vi "DT_With_Multiplexer.vi"() -> ()   [LabVIEW 2012]
doc: "This vi will take data with multiple DT boxes for an arbitrary number of channels either differentially or single ended, depending upon how you have wired the boxes up."
uses:
  Globals/Meas_global.vi
panel:
  out "Waveform Graph":dbl[][](graph)
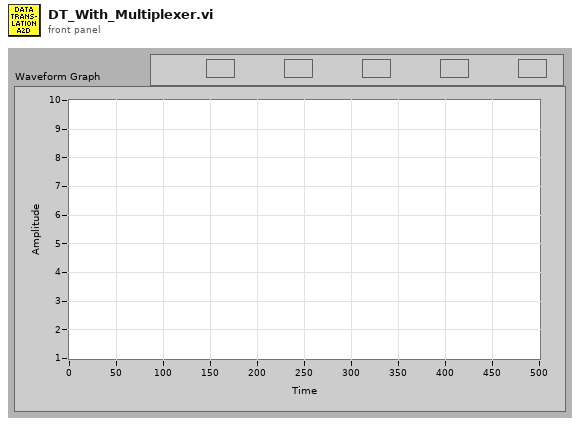
[diagram p1: front panel]
types:
  T1 = typedef "Trigger_Mode.ctl" = enum16{"Free Running", "Start on Trigger", "Trigger Every Block", "Trigger Every Sample"}
  T2 = typedef "LDA_Setup.ctl" = cluster{"dimensions":enum16{"1D", "2D"}, "Analogue Freq Multiplier":dbl}
  T3 = typedef "Ch_and_Spans.ctl" = cluster{"high limit (10V)":sgl, "low limit (-10V)":sgl, "Ch No":i16, "Var name":string, "Use Latest Calib":bool}
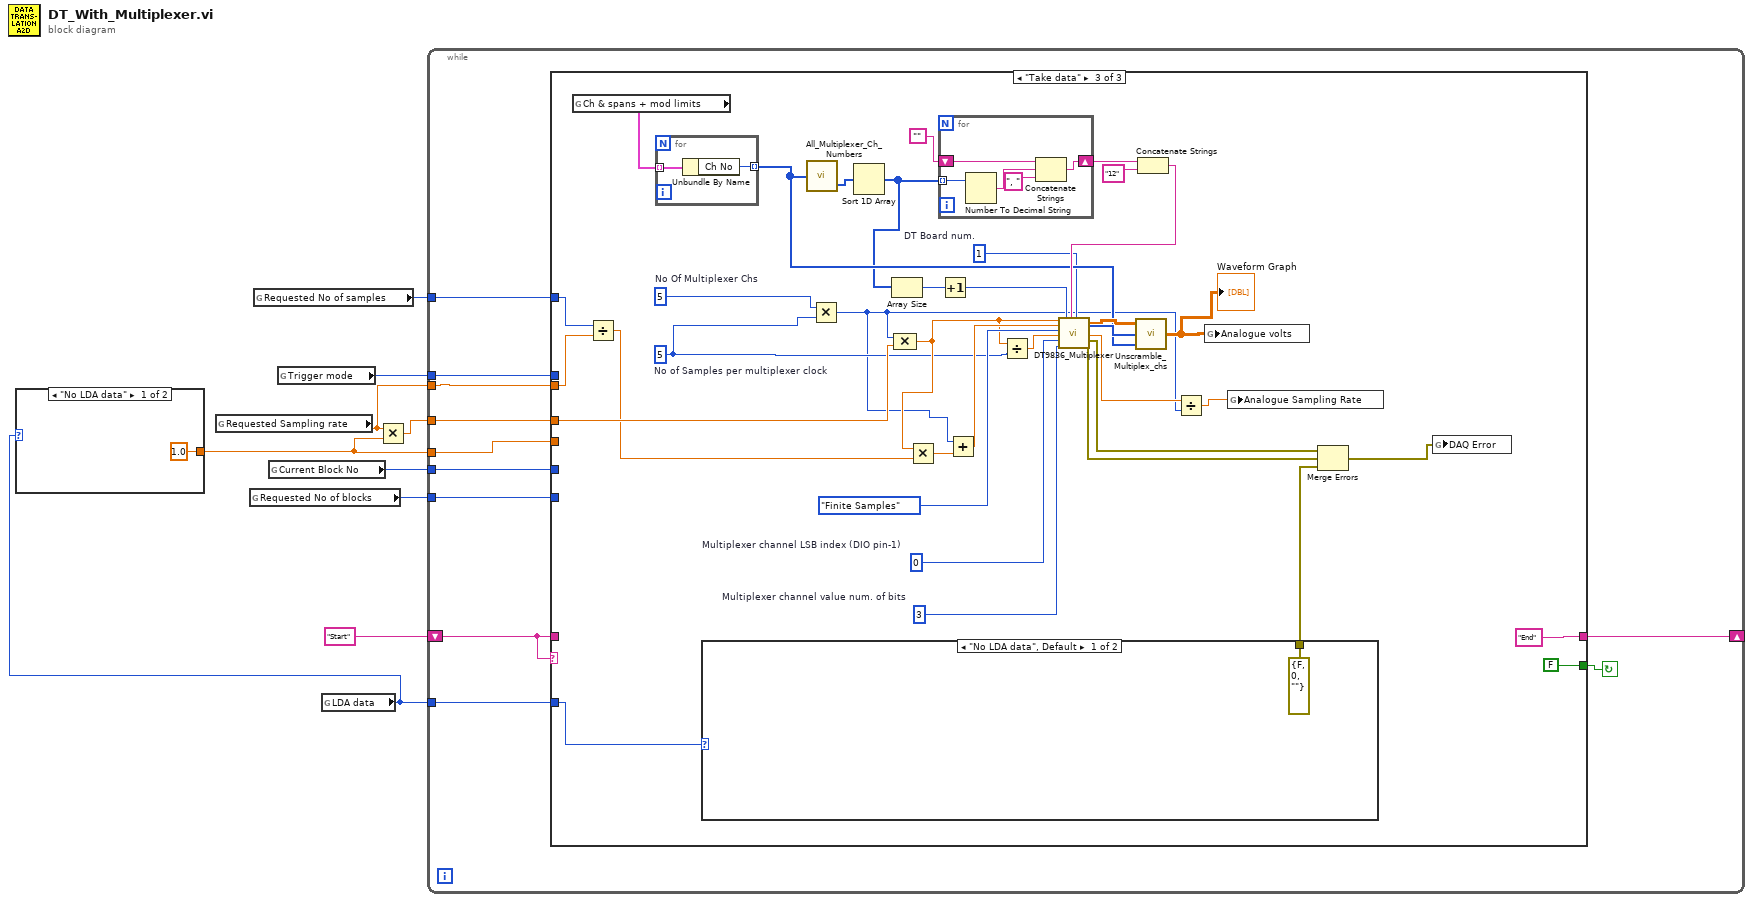
[diagram p0: block diagram]
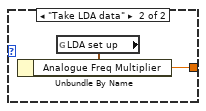
[diagram p2: hidden frame]
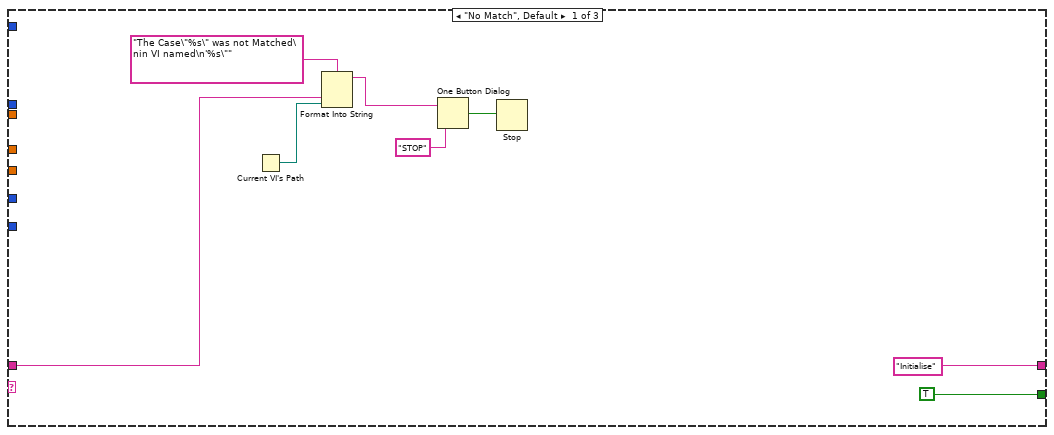
[diagram p3: hidden frame]
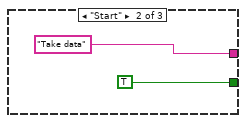
[diagram p4: hidden frame]
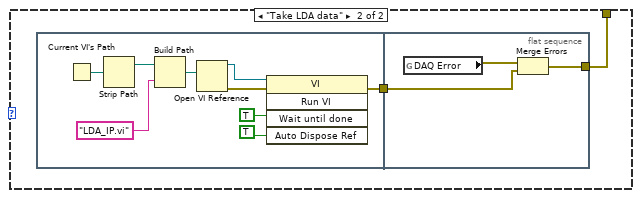
[diagram p5: hidden frame]
diagram:
  n1 = global read "Meas_global.vi" "Requested Sampling rate"() -> (w4:dbl)
  n2 = global read "Meas_global.vi" "Requested No of blocks"() -> (w3:i32)
  n3 = global read "Meas_global.vi" "Requested No of samples"() -> (w8:i32)
  n4 = global read "Meas_global.vi" "Current Block No"() -> (w6:i32)
  n5 = global read "Meas_global.vi" "Trigger mode"() -> (w7:T1)
  n6 = global read "Meas_global.vi" "LDA data"() -> (w1:enum16{"No LDA data", "Take LDA data"})
  n7 = case shown="\"No LDA data\"" w1 {
    tunnel: [1.0 ("Analogue Freq Multiplier") w11] -> w2
    frame "No LDA data" {
    }
    frame "Take LDA data" {
      n8 = global read "Meas_global.vi" "LDA set up"() -> (w12:T2)
      n9 = Unbundle By Name(w12) -> ("Analogue Freq Multiplier"=w11:dbl)
    }
  }
  n10 = Multiply(x=w4, y=w2) -> (x*y=w5:dbl)
  n11 = while {
    shift-left: "Start" -> [w22]
    shift-right: [w23] -> _
    tunnel: w5 -> [w21]
    tunnel: w8 -> [w20]
    tunnel: w6 -> [w19]
    tunnel: w7 -> [w17]
    tunnel: w1 -> [w16]
    tunnel: w2 -> [w15]
    tunnel: w4 -> [w14]
    tunnel: w3 -> [w13]
    stop <- w18 continue-if-true
    n12 = case shown="\"Take data\"" w22 {
      tunnel: ["Initialise" "Take data" "End"] -> w23
      tunnel: w22 -> [w27 _ _]
      tunnel: w21 -> [_ _ w62]
      tunnel: w20 -> [_ _ w61]
      tunnel: w19 -> [_ _ _]
      tunnel: [TRUE TRUE FALSE] -> w18
      tunnel: w17 -> [_ _ _]
      tunnel: w16 -> [_ _ w68]
      tunnel: w15 -> [_ _ _]
      tunnel: w14 -> [_ _ w39]
      tunnel: w13 -> [_ _ _]
      frame "No Match", Default {
        n13 = Current VI's Path() -> (path=w26:path)
        n14 = Format Into String(format string="The Case\"%s\" was not Matched\nin VI named\n'%s\"" ("Format String"), w27, w26) -> (resulting string=w30:string)  [unwired: 2 in, 1 out]
        n15 = One Button Dialog(message=w30, button name ("OK")="STOP") -> (true=w28:bool)
        n16 = Stop(stop? (T)=w28) -> ()
      }
      frame "Start" {
      }
      frame "Take data" {
        w44 = 3  # Multiplexer channel value num. of bits
        w45 = 0  # Multiplexer channel LSB index (DIO pin-1)
        w46 = u32 1  # DT Board num.
        w54 = 5  # No of Samples per multiplexer clock
        w58 = 5  # No Of Multiplexer Chs
        n17 = global read "Meas_global.vi" "Ch & spans + mod limits"() -> (w67:T3[])
        n18 = Divide(x=w61, y=w39) -> (x/y=w60:dbl)
        n19 = for {
          tunnel: w67 -> [w77] mode=indexing
          tunnel: [w76] -> w49 mode=indexing
          n20 = Unbundle By Name(w77) -> ("Ch No"=w76:i16)
        }
        n21 = case shown="\"No LDA data\", Default" w68 {
          tunnel: [errorcluster {"status"=FALSE, "code"=0, "source"=""} ("error IO") w79] -> w41
          frame "No LDA data", Default {
          }
          frame "Take LDA data" {
            n22 = flat-sequence {
              tunnel: [w81] -> w80
              tunnel: w80 -> [w91]
              tunnel: [w90] -> w79
              frame #0 {
                n23 = Current VI's Path() -> (path=w83:path)
                n24 = Strip Path(path=w83) -> (stripped path=w82:path)  [unwired: 1 out]
                n25 = Build Path(base path=w82, name or relative path="LDA_IP.vi") -> (appended path=w84:path)
                n26 = Open VI Reference(vi path=w84) -> (vi reference=w87:refnum<vi>, error out=w88:errorcluster)  [unwired: 5 in]
                n27 = invoke class="VI" method="Run VI"(reference=w87, error in=w88, "Wait until done"=TRUE ("Wait Until Done"), "Auto Dispose Ref"=TRUE ("Wait until done")) -> (error out=w81:errorcluster)  [unwired: 1 in, 4 out]
              }
              frame #1 {
                n28 = global read "Meas_global.vi" "DAQ Error"() -> (w92:errorcluster)
                n29 = Merge Errors(w92, w91) -> (w90:errorcluster)
              }
            }
          }
        }
        n30 = call "All_Multiplexer_Ch_Numbers.vi"("Channel Numbers"=w49) -> ("ADC Ch No"=w38:i16[])  [unwired: 1 out]
        n31 = Multiply(x=w58, y=w54) -> (x*y=w35:i32)
        n32 = Sort 1D Array(array=w38) -> (sorted array=w37:i16[])
        n33 = Array Size(array=w37) -> (size(s)=w48:i32)
        n34 = Compound Arithmetic op=MULTIPLY(w35, w62) -> (w55:dbl)
        n35 = Multiply(x=w55, y=w60) -> (x*y=w59:dbl)
        n36 = for {
          tunnel: w37 -> [w75] mode=indexing
          shift-right: [w71] -> w64
          shift-left: "" -> [w72]
          n37 = Number To Decimal String(number=w75) -> (decimal integer string=w74:string)  [unwired: 1 in]
          n38 = Concatenate Strings(w72, w74, ", " ("string")) -> (w71:string)
        }
        n39 = Increment(x=w48) -> (x+1=w47:i32)
        n40 = Add(x=w35, y=w59) -> (x+y=w57:dbl)
        n41 = Divide(x=w55, y=w54) -> (x/y=w53:dbl)
        n42 = Concatenate Strings(w64, "12" ("string")) -> (w63:string)
        n43 = call "DT9836_Multiplexer.vi"("Sample Freq (Hz)"=w55, "Samples Per Channel"=w57, "Sample Mode"=enum16{"Finite Samples", "Continuous Samples"}."Finite Samples", "Multiplexer cycle freq. (Hz)"=w53, "Multiplexer channel LSB index (DIO pin-1)"=w45, "Multiplexer channel value num. of bits"=w44, "Number Chan to Read"=w47, "Channel list (12 for Digital IO)"=w63, "DT Board num."=w46) -> ("2D volts out"=w51:dbl[][], "Multiplexer channel"=w52:u32[], "Actual Sample Freq"=w36:dbl, "Data acq. final error"=w43:errorcluster, "Clock error"=w42:errorcluster)  [unwired: 6 in]
        n44 = call "Unscramble_Multiplex_chs.vi"("Channel Numbers"=w49, "Multiplex Ch No"=w52, "Voltages"=w51) -> ("Voltage by Req Ch"=w50:dbl[][])
        "Waveform Graph" <- w50
        n45 = Divide(x=w36, y=w35) -> (x/y=w34:dbl)
        n46 = global write "Meas_global.vi" "Analogue volts"(w50) -> ()
        n47 = global write "Meas_global.vi" "Analogue Sampling Rate"(w34) -> ()
        n48 = Merge Errors(w43, w42, w41) -> (w40:errorcluster)
        n49 = global write "Meas_global.vi" "DAQ Error"(w40) -> ()
      }
    }
  }
